vi "5.4.vi"() -> ()   [LabVIEW 2017]
uses:
  <vilib>/measure/NI_MABase.lvlib
panel:
  out "波形图":waveform(dbl)(graph)
  in  "frequency":dbl=10.0 caption="频率" format="%0.2p"
  in  "amplitude":dbl=1.0 caption="幅值" format="%0.2p"
  in  "phase":dbl caption="相位" format="%.2p"
  in  "sampling info":cluster{"Fs":dbl, "#s":dbl}={"Fs"=1000.0, "#s"=1000.0} caption="采样信息" {"Fs" format="%.2p"}
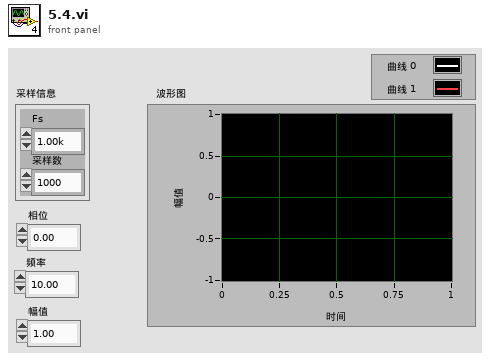
[diagram p1: front panel]
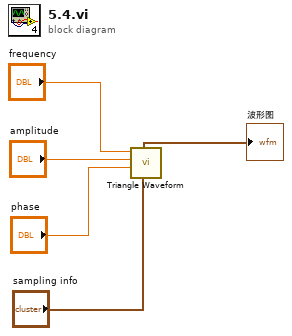
[diagram p0: block diagram]
diagram:
  n1 = call <vilib>:"Triangle Waveform.vi"("sampling info"="sampling info", "phase"="phase", "amplitude"="amplitude", "frequency"="frequency") -> ("signal out"=→"波形图":waveform(dbl))  [unwired: 6 in, 1 out]
